vi "ControlReference.GetReferenceToControl.vi"(8 "error in (no error)":errorcluster, 10 "controlLabelText":string, 11 "referenceToControls in":refnum<vi>[](array[refnum])) -> (0 "error out":errorcluster, 2 "referenceToControl":refnum<vi>, 3 "referenceToControls out":refnum<vi>[](array[refnum]))   [LabVIEW 2019]
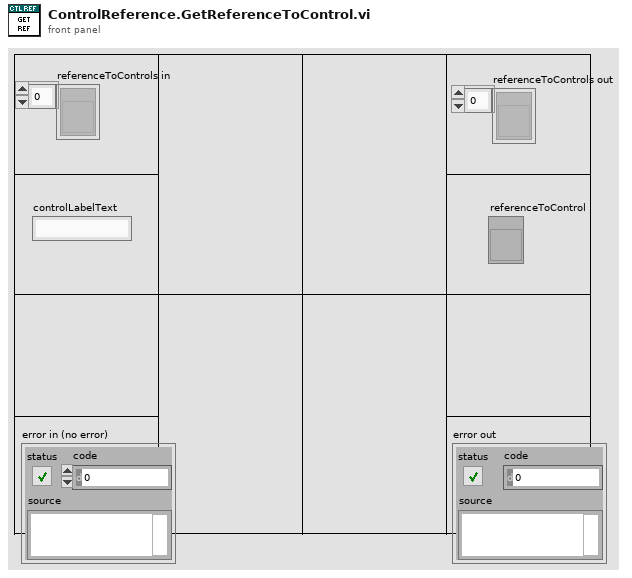
[diagram p1: front panel]
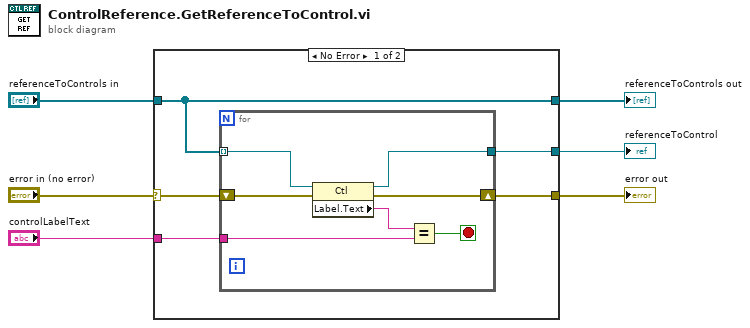
[diagram p0: block diagram]
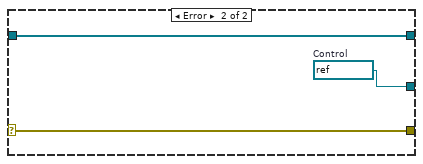
[diagram p2: hidden frame]
diagram:
  n1 = case shown="No Error" "error in (no error)" {
    selector: "error in (no error)" -> [w10 w20]
    tunnel: [w11 w21] -> w4
    tunnel: "referenceToControls in" -> [w11 w21]
    tunnel: [w9 w20] -> w6
    tunnel: "controlLabelText" -> [w8 _]
    tunnel: [w7 w19] -> w1
    frame No Error {
      n2 = for {
        tunnel: w11 -> [w18] mode=indexing
        shift-right: [w16] -> w9
        shift-left: w10 -> [w17]
        tunnel: w8 -> [w13]
        tunnel: [w12] -> w7
        stop <- w15 stop-if-true
        n3 = property class="Ctl"(reference=w18, error in=w17) -> (reference out=w12:refnum<vi>, error out=w16:errorcluster, "Label.Text"=w14:string)
        n4 = Equal?(x=w14, y=w13) -> (x = y?=w15:bool)
      }
    }
    frame Error {
      w19 = refnum<vi> refnum  # Control
    }
  }
  "error out" <- w6
  "referenceToControls out" <- w4
  "referenceToControl" <- w1
